vi "Initialize.vi"(0 "VISA resource name":refnum<visa-resource-name>="TCPIP::192.168.0.2::INSTR", 5 "ID Query (True)":bool=TRUE, 7 "Reset (True)":bool=TRUE, 11 "error in (no error)":errorcluster, 12 "Timeout (10000 ms)":u32=10000) -> (4 "VISA resource name out":refnum<visa-resource-name>, 15 "error out":errorcluster)   [LabVIEW 2020, in "NH Research Regenerative Test Series.lvlib"]
uses:
  NH Research Regenerative Test Series.lvlib
panel:
  out "Model Number":string
  out "Firmware Version":string
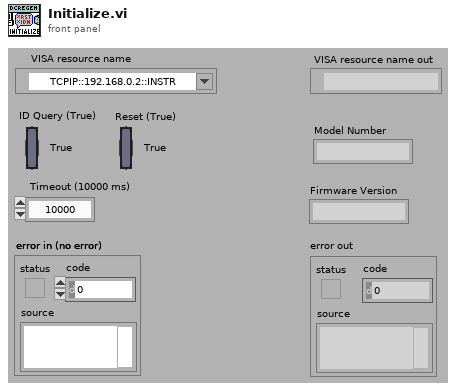
[diagram p1: front panel]
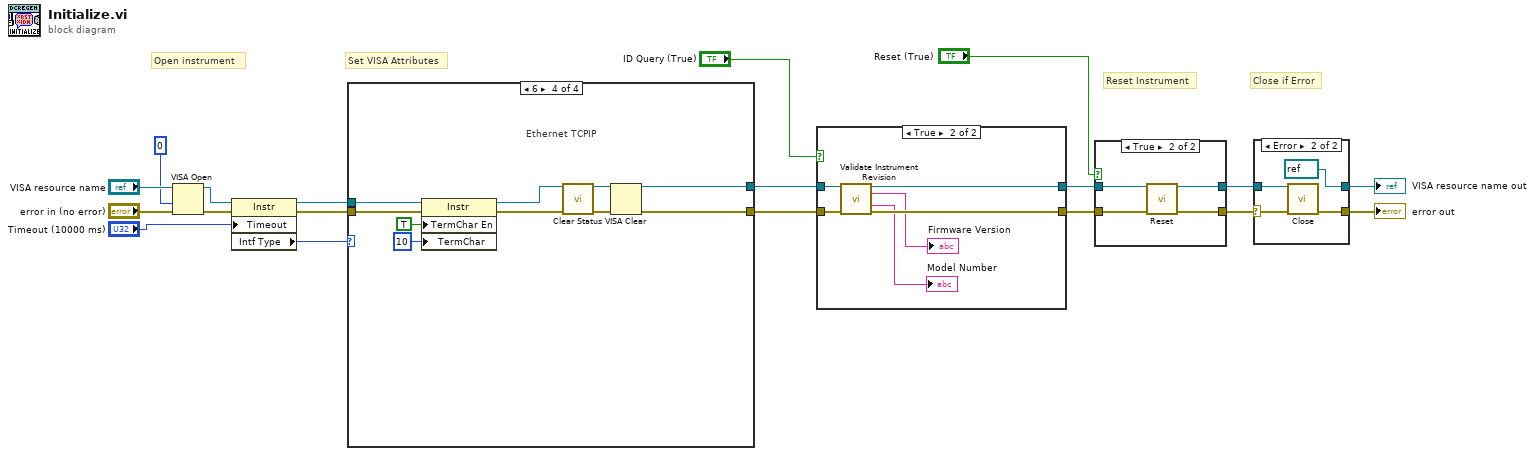
[diagram p0: block diagram]
diagram:
  # "Set VISA Attributes"
  # "Close if Error"
  # "Reset Instrument"
  # "Open instrument"
  n1 = VISA Open(access mode=u32 0, error in (no error)="error in (no error)", VISA resource name="VISA resource name") -> (VISA resource name=w14:refnum<visa-resource-name>, error out=w13:errorcluster)  [unwired: 2 in]
  n2 = property on="Property Node" class="Instr"(reference=w14, error in=w13, "Timeout"="Timeout (10000 ms)") -> (reference out=w8:refnum<visa-resource-name>, error out=w7:errorcluster, "Intf Type"=w6:u16)
  n3 = case shown="6" w6 {
    tunnel: [w21 w22 w24 w34] -> w16
    tunnel: [w20 w23 w25 w33] -> w15
    tunnel: w8 -> [w21 w22 w24 w31]
    tunnel: w7 -> [w20 w23 w25 w27]
    frame Default {
    }
    frame 1 {
      # "GPIB Interface - Not Supported"
    }
    frame 4 {
      # "Serial Interface - Not Supported"
    }
    frame 6 {
      # "Ethernet TCPIP"
      n4 = property on="Property Node" class="Instr"(reference=w31, error in=w27, "TermChar En"=TRUE ("Message Based Settings:Termination Character Enable"), "TermChar"=u8 10 ("Message Based Settings:Termination Character")) -> (reference out=w28:refnum<visa-resource-name>, error out=w26:errorcluster)
      n5 = call "Clear Status.vi"("VISA resource name"=w28, "error in (no error)"=w26) -> ("VISA resource name out"=w32:refnum<visa-resource-name>, "error out"=w35:errorcluster)  [unwired: 12 in]
      n6 = VISA Clear(VISA resource name=w32, error in (no error)=w35) -> (VISA resource name out=w34:refnum<visa-resource-name>, error out=w33:errorcluster)
    }
  }
  n7 = case shown="True" "ID Query (True)" {
    tunnel: w16 -> [w37 w43]
    tunnel: w15 -> [w36 w42]
    tunnel: [w36 w41] -> w3
    tunnel: [w37 w40] -> w2
    frame False {
    }
    frame True {
      n8 = call "Validate Instrument Revision.vi"("VISA resource name"=w43, "error in (no error)"=w42) -> ("VISA resource name out"=w40:refnum<visa-resource-name>, "Firmware Version"=→"Firmware Version":string, "Model Number"=→"Model Number":string, "error out"=w41:errorcluster)  [unwired: 10 in]
    }
  }
  n9 = case shown="True" "Reset (True)" {
    tunnel: w3 -> [w44 w46]
    tunnel: [w44 w48] -> w5
    tunnel: w2 -> [w45 w47]
    tunnel: [w45 w49] -> w10
    frame False {
    }
    frame True {
      n10 = call "Reset.vi"("VISA resource name"=w47, "error in (no error)"=w46) -> ("VISA resource name out"=w49:refnum<visa-resource-name>, "error out"=w48:errorcluster)  [unwired: 12 in]
    }
  }
  n11 = case shown="Error" w5 {
    selector: w5 -> [w50 w53]
    tunnel: w10 -> [w51 w54]
    tunnel: [w51 refnum<visa-resource-name> refnum ("VISA resource name out")] -> w12
    tunnel: [w50 w55] -> w11
    frame No Error {
    }
    frame Error {
      n12 = call "Close.vi"("VISA resource name"=w54, "error in (no error)"=w53) -> ("error out"=w55:errorcluster)  [unwired: 13 in]
    }
  }
  "VISA resource name out" <- w12
  "error out" <- w11
